vi "get folder file name paths list.vi"(8 "error in":errorcluster, 10 "Write output file?":bool, 11 "file search pattern":string="*_P_*") -> (0 "error out":errorcluster, 1 "Records":i32, 2 "Selected folder path":string, 3 "File path names":string[](array[string]))   [LabVIEW 2013]
panel:
  out "Numeric":i32
  out "csv data":string
  out "Part Nums":string[](array[string])
  out "files":i32
  out "Sub-folder files":string[](array[string])
  out "folder names":string[](array[string])
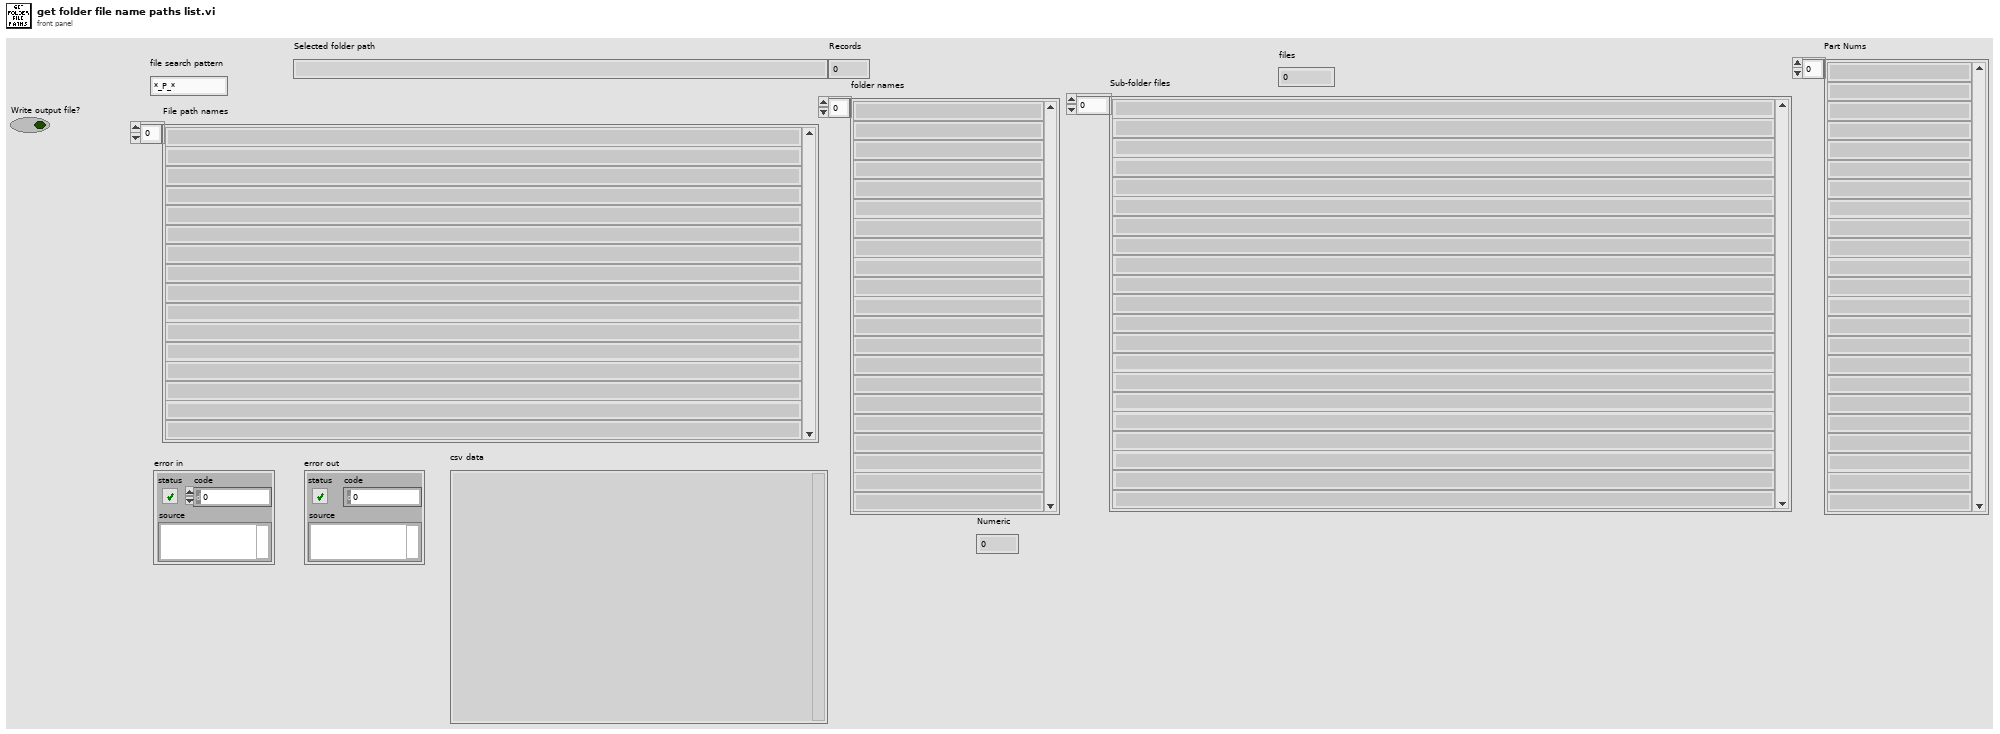
[diagram p1: front panel]
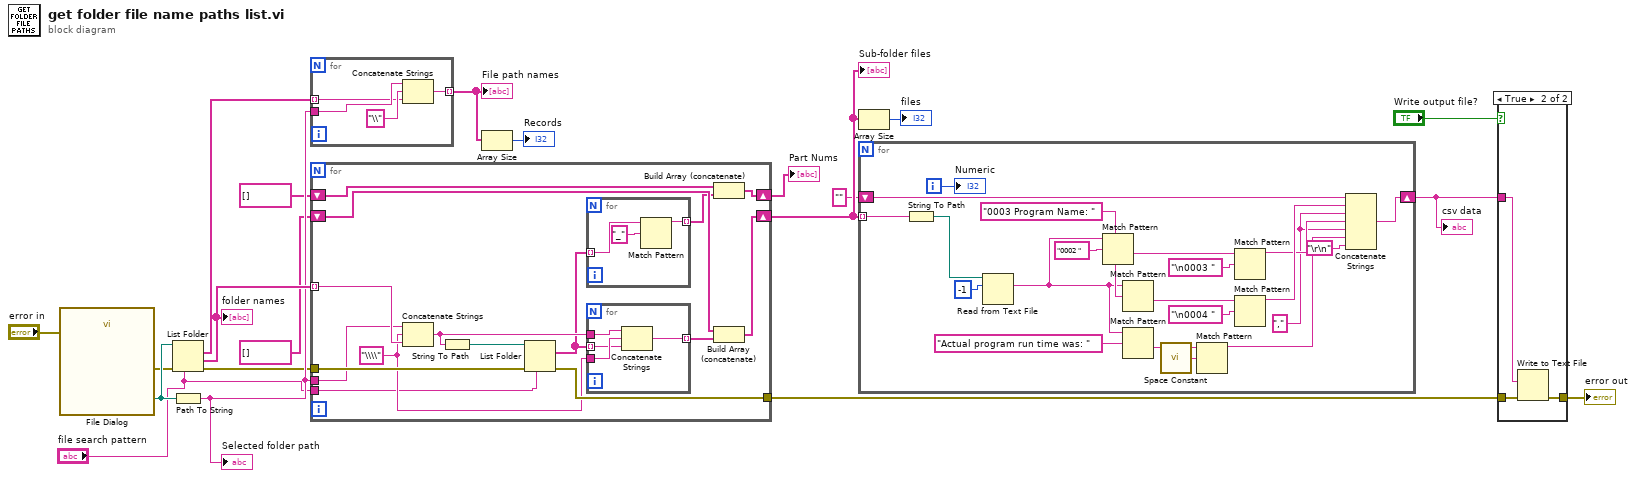
[diagram p0: block diagram]
diagram:
  n1 = call "File Dialog"("error in"="error in") -> ("selected path"=w20:path, "error out"=w17:errorcluster)  [unwired: 11 in, 2 out]
  n2 = List Folder(path=w20, pattern="file search pattern", error in=w17) -> (filenames=w19:string[], folder names=w14:string[], error out=w12:errorcluster)  [unwired: 1 in, 1 out]
  "folder names" <- w14
  n3 = Path To String(path=w20) -> (string=w13:string)
  "Selected folder path" <- w13
  n4 = for {
    tunnel: w19 -> [w22] mode=indexing
    tunnel: w13 -> [w24]
    tunnel: [w21] -> w16 mode=indexing
    n5 = Concatenate Strings(w24, "\\" ("string"), w22) -> (w21:string)
  }
  "File path names" <- w16
  n6 = for {
    tunnel: w14 -> [w39] mode=indexing
    tunnel: w13 -> [w33]
    tunnel: w12 -> [w37]
    shift-right: [w35] -> w7
    shift-left: string[] [] -> [w36]
    tunnel: [w34] -> w4
    shift-right: [w26] -> w8
    shift-left: string[] [] -> [w28]
    tunnel: "file search pattern" -> [w25]
    w32 = "\\\\" ("string")
    n7 = Concatenate Strings(w33, w32, w39) -> (w30:string)
    n8 = String To Path(string=w30) -> (path=w38:path)
    n9 = List Folder(path=w38, pattern=w25, error in=w37) -> (filenames=w29:string[], error out=w34:errorcluster)  [unwired: 1 in, 2 out]
    n10 = for {
      tunnel: w29 -> [w42] mode=indexing
      tunnel: [w40] -> w27 mode=indexing
      n11 = Match Pattern(string=w42, regular expression="_") -> (before substring=w40:string)  [unwired: 1 in, 3 out]
    }
    n12 = for {
      tunnel: w29 -> [w45] mode=indexing
      tunnel: w32 -> [w46]
      tunnel: [w44] -> w31 mode=indexing
      tunnel: w30 -> [w43]
      n13 = Concatenate Strings(w43, w46, w45) -> (w44:string)
    }
    n14 = Build Array (concatenate)(w28, w27) -> (w26:string[])
    n15 = Build Array (concatenate)(w36, w31) -> (w35:string[])
  }
  "Sub-folder files" <- w7
  "Part Nums" <- w8
  n16 = Array Size(array=w16) -> (size(s)=→"Records":i32)
  n17 = Array Size(array=w7) -> (size(s)=→"files":i32)
  n18 = for {
    tunnel: w7 -> [w67] mode=indexing
    shift-right: [w48] -> w5
    shift-left: "" -> [w49]
    i -> [w47]
    w53 = "," ("string")
    n19 = String To Path(string=w67) -> (path=w66:path)
    n20 = Read from Text File(file (use dialog)=w66, count=-1) -> (text=w58:string)  [unwired: 2 in, 3 out]
    n21 = Match Pattern(string=w58, regular expression="0002 ") -> (after substring=w61:string)  [unwired: 1 in, 3 out]
    n22 = Match Pattern(string=w58, regular expression="0003 Program Name: ") -> (after substring=w59:string)  [unwired: 1 in, 3 out]
    n23 = Match Pattern(string=w58, regular expression="Actual program run time was: ") -> (after substring=w56:string)  [unwired: 1 in, 3 out]
    n24 = call <vilib>:"Space Constant.vi"() -> ("String"=w52:string)
    n25 = Match Pattern(string=w56, regular expression=w52) -> (before substring=w51:string)  [unwired: 1 in, 3 out]
    n26 = Match Pattern(string=w61, regular expression="\n0003 ") -> (before substring=w54:string)  [unwired: 1 in, 3 out]
    n27 = Match Pattern(string=w59, regular expression="\n0004 ") -> (before substring=w55:string)  [unwired: 1 in, 3 out]
    n28 = Concatenate Strings(w49, w55, w53, w54, w53, w51, "\r\n") -> (w48:string)
    "Numeric" <- w47
  }
  "csv data" <- w5
  n29 = case shown="True" "Write output file?" {
    tunnel: w5 -> [_ w71]
    tunnel: w4 -> [w68 w70]
    tunnel: [w68 w69] -> w3
    frame False {
    }
    frame True {
      n30 = Write to Text File(text=w71, error in=w70) -> (error out=w69:errorcluster)  [unwired: 2 in, 2 out]
    }
  }
  "error out" <- w3
